vi "SetOrderedList.vi"(8 "error in (no error)":errorcluster, 10 "OrderedList":refnum<class "Collection.lvclass">, 11 "OrderedList in":refnum<class "OrderedList.lvclass">) -> (0 "error out":errorcluster, 3 "OrderedList out":refnum<class "OrderedList.lvclass">)   [LabVIEW 2021, in "Markdown.lvlib" / "OrderedList.lvclass"]
uses:
  OrderedList.lvclass
  Collection/Collection.lvclass
  OrderedList.lvclass/OrderedList.ctl
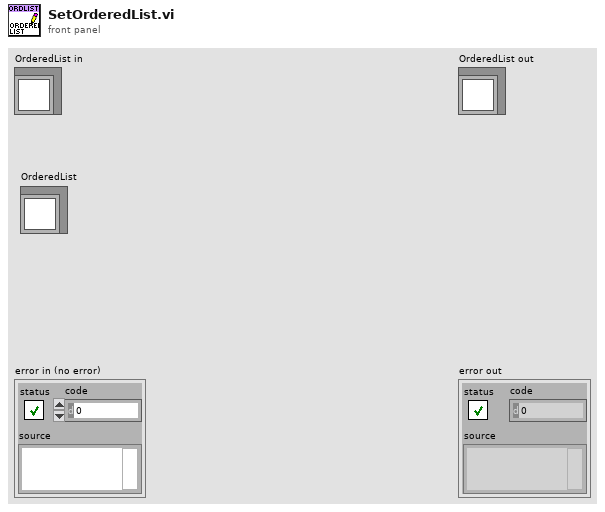
[diagram p1: front panel]
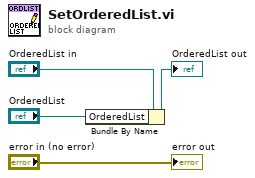
[diagram p0: block diagram]
diagram:
  n1 = Bundle By Name(cluster="OrderedList in", "OrderedList"="OrderedList") -> (→"OrderedList out":refnum<class "OrderedList.lvclass">)
  "error out" <- "error in (no error)"
